vi "dfd_nMAC_SubNwLoad.vi"(0 "initIdx":fxp<+,16,16>, 3 "load":bool, 4 "step":fxp<+,16,16>) -> (6 "wrapZero?":bool, 7 "idxOut":fxp<+,16,16>)   [LabVIEW 2017]
uses:
  <vilib>/rvi/FXPMathLib/basic elements/FxpAddSub/XNode/nifxpmath_AddSub.xnode
  <vilib>/rvi/FXPMathLib/sim/FxpSim.dll
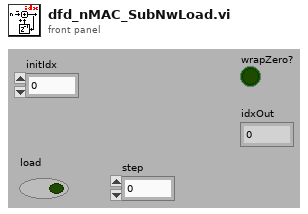
[diagram p1: front panel]
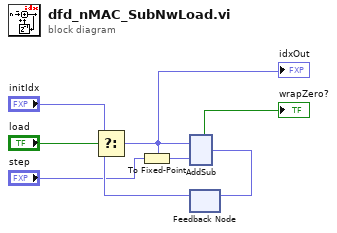
[diagram p0: block diagram]
diagram:
  n1 = feedback #1() -> (w5:fxp<+,16,16>)  [unwired: 1 out]
  n2 = Select(t="initIdx", s="load", f=w5) -> (s? t:f=w1:fxp<+,16,16>)
  "idxOut" <- w1
  n3 = To Fixed-Point(fixed-point type=w1, number="step") -> (fixed-point=w2:fxp<+,16,16>)
  n4 = xnode "AddSub"("x"=w1, "y"=w2) -> ("s"=w6:fxp<+,16,16>, "borrow-out"=→"wrapZero?":bool)
  n5 = feedback-in #1(w6) -> ()
